vi "globalVarSD.vi"() -> ()   [LabVIEW 2018]
panel:
  out "Init DAQmx tasks":bool
  out "Init detector":bool
  out "Init DL":bool
  out "Init success":bool
  in  "path alarm sound":path=path "G:/SD/TRANCON/sounds/swgzq-rkyg3.wav"
  in  "accuracy":string="%.4f"
  out "Break measurement":bool
  in  "wavelength fix index":i16
  in  "sigma":dbl
  in  "clean mode":enum32{"delete", "approximate"}(radio)
  in  "Old/New":bool
  in  "Application path":path
  in  "Slash":string="\\"
  in  "# points":i32
  in  "Real zero":dbl
  in  "Cut ON/OFF":bool
  in  "BasePath":path
  in  "Type of detection":enum32{"IR detection", "UV-vis detection"}(radio)
  in  "deltaT":dbl
  in  "delay0":dbl
  in  "pixel+":i32
  in  "pixel-":i32
  in  "Log":bool
  in  "error min":dbl=0.0001
  in  "shift":i32
  out "Dev":bool
  out "wavelengths":dbl[](array[numeric])=[1.74695840294851, 1.73947371440581, 1.73199263543554, 1.72451569505241, 1.71704336159476, 1.70957618537218, 1.70211465103603, 1.69465931938089, 1.68721070135242, 1.6797693560201301, 1.67233583286395, 1.66491067290181, 1.65749448123694, 1.65008777499183, 1.64269118936313, 1.63530526816863, 1.62793059787024, 1.62056782564518, 1.6132174869458, 1.60588021624955, 1.59855664914169, 1.59124734594406, 1.58395293766588, 1.57667410341541, 1.56941139768648, 1.56216544706426, 1.55493690232794, 1.54772642715279, 1.54053459790541, 1.53336204673031, 1.5262094059754, 1.5190773076058, 1.51196639712882, 1.50487731519191, 1.49781065537266, 1.49076704050463, 1.48374708968683, 1.4767514175569, 1.4697806335417, 1.46283534108578, 1.45591613685827, 1.44902362355376, 1.4421584350399, 1.43532109764276, 1.42851217454608, 1.42173221797025, 1.41498176826326, 1.40826153129896, 1.40157188671621, 1.39491332390898, 1.38828653993869, 1.38169189429006, 1.37512987969607, 1.36860110805257, 1.3621058521608, 1.35564479016035, 1.3492181722474, 1.34282652069934, 1.33647029749548, 1.33014974492859, 1.32386540164977, 1.31761765329026, 1.31140674343692, 1.30523303537283, 1.29909687508932, 1.29299859208834, 1.28693855623105, 1.28091695705859, 1.27493406221769, 1.26899011878883, 1.26308544991285, 1.25722022338053, 1.25139461273802, 1.2456087796279, 1.23986286216394, 1.23415717021322, 1.22849182981838, 1.2228667403288, 1.2172823138312, 1.21173844101154, 1.20623526099378, 1.20077284844751, 1.19535128728291, 1.18997039739273, 1.18463066565183, 1.17933166025863, 1.174073424022, 1.16885619951437, 1.16367983262934, 1.15854420056361, 1.15344927142328, 1.14839499472779, 1.14338130122296, 1.13840810270664, 1.13347529186764, 1.12858274213783, 1.12373030755832, 1.11891782265939, 1.1141453578523, 1.10941267699039, 1.10471941530734, 1.10006545035942, 1.0954509959156, 1.09087526672658, 1.0863386046025, 1.08184037921328, 1.07738075829889, 1.07295905446028, 1.0685757295472, 1.06422989459505, 1.05992154623097, 1.05565074890564, 1.05141685513876, 1.0472196667672, 1.04305897437087, 1.03893469695662, 1.03484651523027, 1.03079405980805, 1.02677707479348, 1.02279529322078, 1.01884843710765, 1.01493621751393, 1.0110584683138, 1.0072149741535, 1.00340527047478, 0.999629026799409, 0.995885902045937, 0.99217596598108, 0.98849879844413, 0.984853757374839, 0.981241054344726, 0.977660158822735, 0.974110590515482, 0.970592605892286, 0.967105210684661, 0.963648839619437, 0.960222603595605, 0.956826487302473, 0.953460345239886, 0.950123391218081, 0.946815901262915, 0.943537424146781, 0.940287407694674, 0.937065621602715, 0.933872182979098, 0.930706610328418, 0.927568480301523, 0.924457544150809, 0.921373548867979, 0.918316237235768, 0.915285347880829, 0.912280615327582, 0.9093017700531, 0.906348538542966, 0.903420643348089, 0.900517803142482, 0.897639732781836, 0.894786143363061, 0.891956742284595, 0.889151695015634, 0.886370451849697, 0.88361257891826, 0.880877770049898, 0.878166234404625, 0.875477603375355, 0.872811181317668, 0.87016718058367, 0.867545430389945, 0.864945008341113, 0.862366773424345, 0.859809471799701, 0.857273487959592, 0.854758299394799, 0.852263819576187, 0.849789719421444, 0.847335982951904, 0.844901929890081, 0.842488162930783, 0.840093417182113, 0.837718515604053, 0.835362615919645, 0.833025256625637, 0.830707311695789, 0.828407649933811, 0.826126036965772, 0.823862809877985, 0.821617722160325, 0.819390181428017, 0.817180036573831, 0.814987181869723, 0.812812007239723, 0.810653714195849, 0.808512147956872, 0.806387152922779, 0.804278572689575, 0.802186250064211, 0.800110027079448, 0.798049745008728, 0.796005244381085, 0.793976454114127, 0.791963086287712, 0.789964959427523, 0.787981911065323, 0.786013831173131, 0.784060630502893, 0.78212207538586, 0.780198000931301, 0.778288241637713, 0.776392631407606, 0.774511003562155, 0.772643190855895, 0.770789025491363, 0.768948339133666, 0.767121449826945, 0.765307967824209, 0.763507516369203, 0.761719925215525, 0.759945023646196, 0.7581833910296, 0.756434390087585, 0.754697623970222, 0.752972920289276, 0.751261192560027, 0.749561354164361, 0.74787311902268, 0.746197142709487, 0.744533015644908, 0.742880029696423, 0.741239027402037, 0.739609387275517, 0.737990423420732, 0.73638361200569, 0.734787227071191, 0.733201926757378, 0.73162764208114, 0.730063551411954, 0.728510886679627, 0.726967845048158, 0.725436176344851, 0.723913978581447, 0.722402723949191, 0.720900885935728, 0.719409739902714, 0.717927776193409, 0.71645643229521, 0.714993856203966, 0.713542007036553, 0.712098780852969, 0.710665667995441, 0.709241510995812, 0.707826617136283, 0.706421219857516, 0.705024166639125, 0.703637106868306, 0.702258385108918, 0.700888369872632, 0.699527668337694, 0.698175030143386, 0.696831212067962, 0.695496163510531, 0.694169015078566, 0.692850439115762, 0.691540448540173, 0.690238194392353, 0.68894390353484, 0.687658374393696, 0.686380417545913, 0.685109988189973, 0.68384778746451, 0.682593529592659, 0.681346634578122, 0.680107057481696, 0.678875371772439, 0.677651411261084, 0.676434603603688, 0.675224903742191, 0.674022266593929, 0.672827515950317, 0.671639819004719, 0.670459019270995, 0.66928507156971, 0.668117930701417, 0.666957767455301, 0.665804889055705, 0.664658651647345, 0.663519009955227, 0.662385918688791, 0.661259332542666, 0.660139206197413, 0.659025494320265, 0.657918577745861, 0.656818087211363, 0.655723844942282, 0.654635805560979, 0.653553923680618, 0.652478153905886, 0.651408450833686, 0.65034476905383, 0.649287063149737, 0.648235287699102, 0.647189397274565, 0.6461493464444, 0.645115089773149, 0.644086581822294, 0.643063777150895, 0.642046630316235, 0.641035095874451, 0.640029128381159, 0.639028682392086, 0.63803371246365, 0.6370441731536, 0.636060019021599, 0.635081204629804, 0.634107684543462, 0.633139413331478, 0.632176345566988, 0.631218435827905, 0.630265638697489, 0.629317908764871, 0.628375200625596, 0.627437468882152, 0.626504668144487, 0.625576753030516, 0.624653678166628, 0.623735398188169, 0.622821867739936, 0.621913041476642, 0.62100892535674, 0.620109953829607, 0.61921558033413, 0.618325759554615, 0.617440446187314, 0.616559594940844, 0.61568316053661, 0.614811097709209, 0.613943361206831, 0.613080378184452, 0.612221994630098, 0.611367831427453, 0.610517843366502, 0.60967198525252, 0.60883021190643, 0.60799247816513, 0.607159693604442, 0.60633093309446, 0.605506106395553, 0.604685168394393, 0.603868073995068, 0.60305511142711, 0.602246732258074, 0.601442091036539, 0.6006411427212, 0.599843842289426, 0.599050453455946, 0.598261610552242, 0.597476310031922, 0.596694506931211, 0.595916156306054, 0.595142093000695, 0.594371942537607, 0.593605139217181, 0.592841638157853, 0.592081906172738, 0.591326408617177, 0.590574108124154, 0.58982495987703, 0.589079419713967, 0.588338078537831, 0.587599784549585, 0.586864492999568, 0.586133005237403, 0.585405324564155, 0.584680541417083, 0.583958611115143, 0.5832410364252, 0.582526521056125, 0.581814753770653, 0.581106377109973, 0.58040188911896, 0.579700044555559, 0.579000804083577, 0.578306103301326, 0.577613941398089, 0.576924273860396, 0.576238621805796, 0.575555902738057, 0.574875573645619, 0.574198903353956, 0.573525387538455, 0.572854157418386, 0.572186407197363, 0.571521855295781, 0.570859484920937, 0.570200593127219, 0.569544766049075, 0.56889101644063, 0.56824092148275, 0.567593580387639, 0.566948212816984, 0.566306853158223, 0.565667759457371, 0.565030744389789, 0.564397849608573, 0.563766764965671, 0.563138393001049, 0.562513372853575, 0.561890059184882, 0.561270268935877, 0.560652885480491, 0.560037363089153, 0.559425835098158, 0.558815850645196, 0.558208818010672, 0.557604554961745, 0.557001744243597, 0.55640312797365, 0.555805892569102, 0.555211479804027, 0.554619757339678, 0.554029520629567, 0.553443236604538, 0.552858171035084, 0.552276240638747, 0.551696479889713, 0.551118679771488, 0.550544149465713, 0.549970675460912, 0.549401090190914, 0.548832713227076, 0.548267212547523, 0.547703858369913, 0.547142427072201, 0.546584021469991, 0.5460266443561, 0.545473113162201, 0.544920358432839, 0.544371044135748, 0.543823030776167, 0.543277725134077, 0.542734379095834, 0.542193066954772, 0.541654314231999, 0.541116980449427, 0.540582747078486, 0.54004937652346, 0.539519588582563, 0.538990239190229, 0.538464749744689, 0.53793971315779, 0.537418141618218, 0.53689734402556, 0.53637967530906, 0.53586304293919, 0.535349261975299, 0.534836721095929, 0.534326812826771, 0.533818289744137, 0.533312239124593, 0.532807660182776, 0.532305452180648, 0.531804743760851, 0.531306363357019, 0.530809451876789, 0.530314884065384, 0.529821695977794, 0.529330925766354, 0.528841387559125, 0.528354399968765, 0.527868438163348, 0.527385218228913, 0.526902759379507, 0.526423292149745, 0.525944262842272, 0.525468533379988, 0.524992860231003, 0.524520853613227, 0.52404884699545, 0.52358016458692, 0.523111865905063, 0.522646378081368, 0.522181772441391, 0.521719405918609, 0.521258478441176, 0.52079915996126, 0.520341895781911, 0.519885552111302, 0.519431936380601, 0.518978494308777, 0.518528512192482, 0.518078530076188, 0.517631535209674, 0.517185171888899, 0.516740917459748, 0.516298158131117, 0.51585657100424, 0.515417400880057, 0.514978407937087, 0.514542812245489, 0.514107216553891, 0.513674304368112, 0.513242268353238, 0.512811789417832, 0.512383298339977, 0.511955179591973, 0.511530218727756, 0.511105257863537, 0.510682941755925, 0.510261496398444, 0.509841379687589, 0.509423435146592, 0.509005490605594, 0.508590986409599] format="%0.3f"
  in  "# d'acquisition par point":u32
  in  "Seuil SC Ref":dbl
  in  "Seuil SC Sig":dbl
  in  "Pixel test":u32
  in  "Nombre d'acquisition par point (réglage)":u32
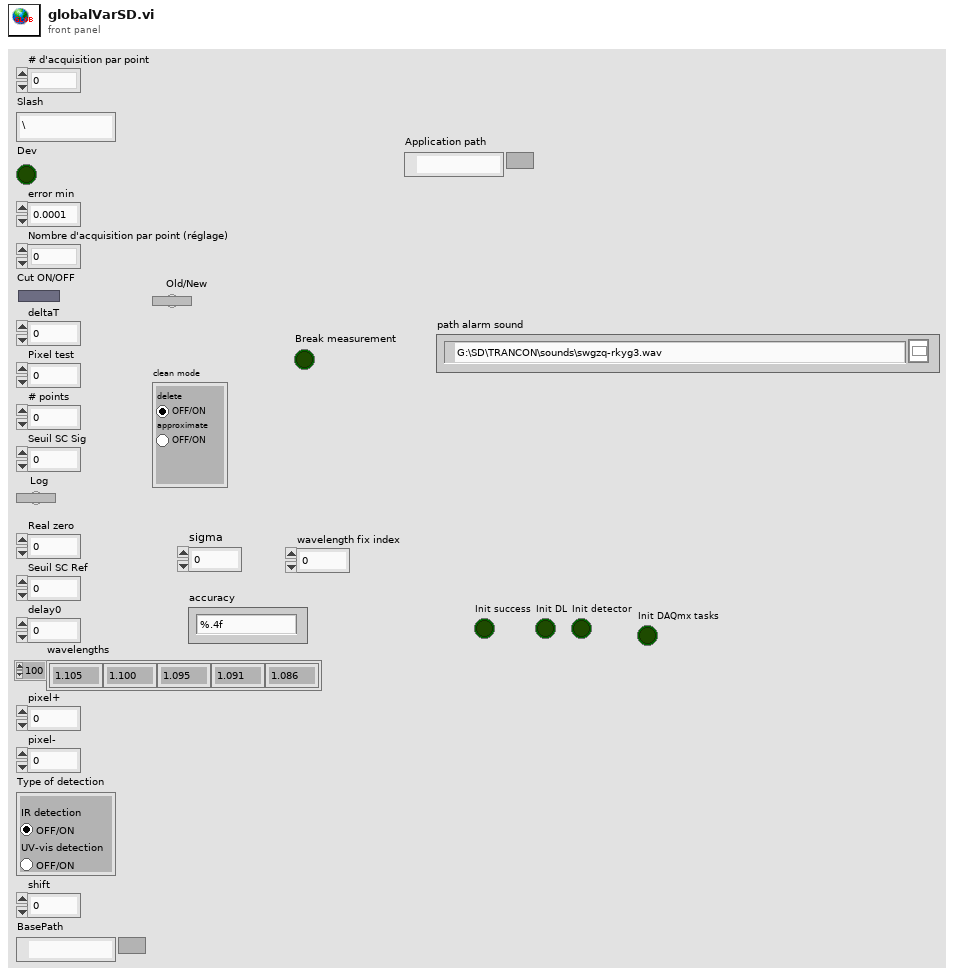
[diagram p1: front panel]
diagram:
